vi "Sub Initialize.vi"(8 "error in (no error)":errorcluster, 11 "Pulse Recorder in":refnum<class "Pulse Recorder.lvclass">) -> (0 "error out":errorcluster, 2 "Initialize Result":refnum<class "Acquired Result.lvclass">, 3 "Pulse Recorder out":refnum<class "Pulse Recorder.lvclass">)   [LabVIEW 2016, in "Pulse Recorder.lvclass"]
uses:
  Pulse Recorder.lvclass
  C:/github/Measure_core/Measure Object/Measure Object.lvclass
  Results/Acquired Result/Acquired Result.lvclass
  Measure Object/Measure Object.lvclass/Measure Object.ctl
  NHMFL_Core/Libraries/Instruments/Pulse Driver/Pulse Driver.lvclass/Pulse Driver.ctl
  NHMFL_Core/Libraries/Instruments/Instrument Driver/Instrument Driver.lvclass/Instrument Driver.ctl
  Measure Object/Read Name.vi
  NHMFL_Core/Libraries/Instruments/Pulse Driver/Write User Configuration.vi
  NHMFL_Core/Libraries/Instruments/Instrument Driver/Write Recorder name.vi
  NHMFL_Core/Libraries/Instruments/Pulse Driver/Pulse Driver.lvclass
  C:/github/NHMFL_Core/Libraries/Instruments/Instrument Driver/Instrument Driver.lvclass
  Read Pulse driver.vi
  Read Pulse Recorder Configuration.vi
  Write Pulse driver.vi
  Instrument Recorders/Instrument Recorder/Instrument Recorder.lvclass
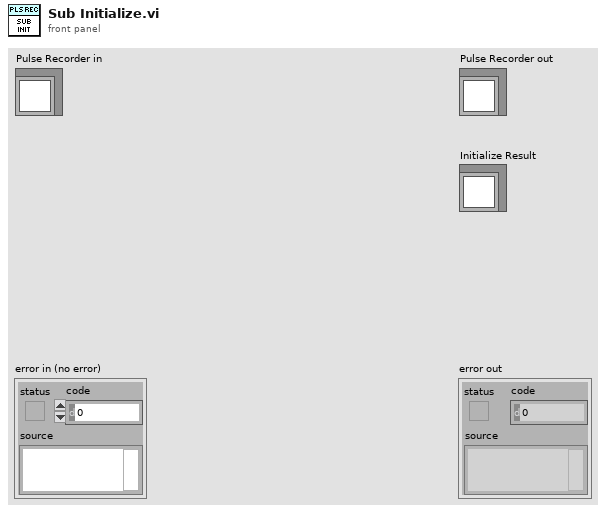
[diagram p1: front panel]
types:
  T1 = typedef "Pusle Driver Configuration.ctl" = cluster{"Pre-trigger duration":dbl, "Post-trigger duration":dbl, "Rate":dbl, "Ranges":dbl[], "Re-name channels":string[], "Active channels":string, "External clock":bool}
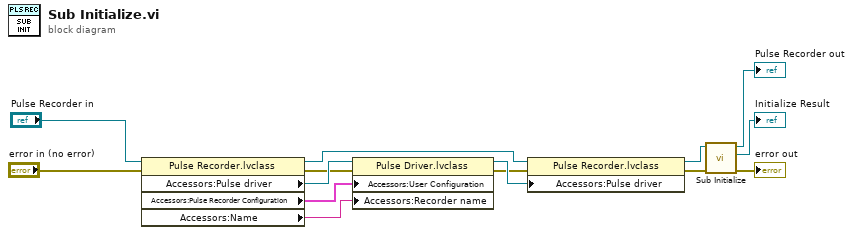
[diagram p0: block diagram]
diagram:
  n1 = property class="Pulse Recorder.lvclass"(reference="Pulse Recorder in", error in="error in (no error)") -> (reference out=w11:refnum<class "Pulse Recorder.lvclass">, error out=w12:errorcluster, "Accessors:Pulse driver"=w13:refnum<class "Pulse Driver.lvclass">, "Accessors:Pulse Recorder Configuration"=w9:T1, "Accessors:Name"=w8:string)
  n2 = property class="Pulse Driver.lvclass"(reference=w13, error in=w12, "Accessors:User Configuration"=w9, "Accessors:Recorder name"=w8) -> (reference out=w5:refnum<class "Pulse Driver.lvclass">, error out=w2:errorcluster)
  n3 = property class="Pulse Recorder.lvclass"(reference=w11, error in=w2, "Accessors:Pulse driver"=w5) -> (reference out=w6:refnum<class "Pulse Recorder.lvclass">, error out=w1:errorcluster)
  n4 = call-parent "Sub Initialize.vi"("error in (no error)"=w1, "Instrument Recorder in"=w6) -> ("error out"=→"error out":errorcluster, "Initialize Result"=→"Initialize Result":refnum<class "Acquired Result.lvclass">, "Instrument Recorder out"=→"Pulse Recorder out":refnum<class "Pulse Recorder.lvclass">)  [unwired: 7 in]
